vi "Add to error queue.vi"(8 "error in (no error)":errorcluster) -> (0 "error out":errorcluster)   [LabVIEW 2020]
uses:
  Error log.ctl
panel:
  out "internal error out":errorcluster
  # "For debugging only"
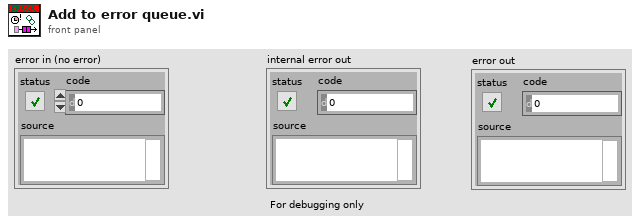
[diagram p1: front panel]
types:
  T1 = typedef "Error log.ctl" = cluster{timestamp, string[], "error in (no error)":errorcluster}
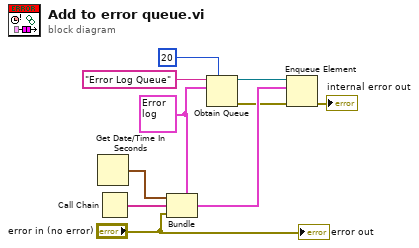
[diagram p0: block diagram]
diagram:
  w7 = T1 {timestamp(0 s since 1904-01-01), [], "error in (no error)"={"status"=FALSE, "code"=0, "source"=""}}
  n1 = Get Date/Time In Seconds() -> (seconds since 1Jan1904=w2:timestamp)
  n2 = Call Chain() -> (call chain=w1:string[])
  n3 = Bundle(cluster=w7, w2, w1, "error in (no error)"="error in (no error)") -> (w6:T1)
  n4 = Obtain Queue(max queue size (-1, unlimited)=20, name (unnamed)="Error Log Queue", element data type=w7) -> (queue out=w8:refnum<queue>, error out=w5:errorcluster)  [unwired: 2 in, 1 out]
  n5 = Enqueue Element(queue=w8, element=w6, error in (no error)=w5) -> (error out=→"internal error out":errorcluster)  [unwired: 1 in, 2 out]
  "error out" <- "error in (no error)"
